vi "Trigger FXP(+,-,18,1).vi"(0 "data A":fxp<+/-,18,1>[](array[numeric])=[0.0, 0.0], 1 "reset":bool, 2 "trigger.ready for reference":bool, 5 "data B":fxp<+/-,18,1>[](array[numeric])=[0.0, 0.0], 7 "input valid":bool, 9 "trigger.A":T9, 11 "trigger.B":T8, 12 "trigger.combination type":T11=enum."A", 13 "rearm delay":u16=2) -> (4 "timestamps":T2, 6 "trigger.out":T10, 8 "overflow":bool, 10 "trigger Source":T1)   [LabVIEW 2021]
uses:
  FPGA Interface Typedefinitions/Trigger Combination Type.ctl
  <instrlib>/_niInstr/Types/v1/Shared/Public/Input Triggers.ctl
  SubVIs/Types/Trigger Type.ctl
  <instrlib>/_niInstr/Data Trigger/v1/Shared/Public/Level Configuration FXP(+-,18,1).ctl
  <instrlib>/_niInstr/Data Trigger/v1/Shared/Public/Level Configuration Trigger When.ctl
  <instrlib>/_niInstr/Data Trigger/v1/Shared/Public/Edge Configuration FXP(+-,18,1).ctl
  <instrlib>/_niInstr/Data Trigger/v1/Shared/Public/Edge Configuration Trigger Slope.ctl
  <instrlib>/_niInstr/Multirecord Acquisition/Interface/v1/FPGA/Public/Timestamp.ctl
  Controls/Clust/TrigSource.ctl
  <instrlib>/_niInstr/Data Trigger/v1/FPGA/Private/Trigger/Level FXP(+-,18,1)xNspc.vi
  <instrlib>/_niInstr/Data Trigger/v1/FPGA/Private/Trigger/Edge FXP(+-,18,1)xNspc.vi
  Trigger Interpolation/Trigger Interpolation FXP(+,-,18,1)x2spc.vi
  <instrlib>/_niInstr/Basic Elements/v1/FPGA/Private/D Latch U16.vi
  <instrlib>/_niInstr/Types/v1/Shared/niInstr Types v1 Shared.lvlib
  <instrlib>/_niInstr/Basic Elements/v1/FPGA/niInstr Basic Elements v1 FPGA.lvlib
  <instrlib>/_niInstr/Data Trigger/v1/FPGA/niInstr Data Trigger v1 FPGA.lvlib
  <instrlib>/_niInstr/Multirecord Acquisition/Interface/v1/FPGA/niInstr Multirecord Acquisition v1 FPGA.lvclass
  <instrlib>/_niInstr/Data Trigger/v1/Shared/niInstr Data Trigger v1 Shared.lvlib
  FPGA Interface Typedefinitions/FPGA Interface Typedefinitions.lvlib
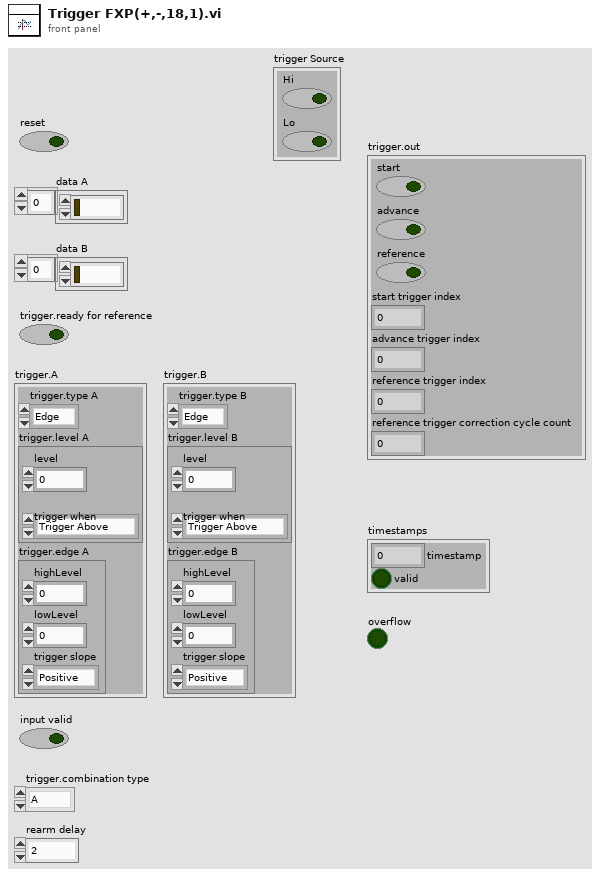
[diagram p1: front panel]
types:
  T1 = typedef "TrigSource.ctl" = cluster{"Hi":bool, "Lo":bool}
  T2 = typedef "niInstr Multirecord Acquisition v1 FPGA.lvclass/Timestamp.ctl" = cluster{"timestamp":u64, "valid":bool}
  T3 = typedef "Trigger Type.ctl" = enum16{"Edge", "Level", "Custom"}
  T4 = typedef "niInstr Data Trigger v1 Shared.lvlib/Level Configuration FXP(+-,18,1).ctl" = cluster{"level":fxp<+/-,18,5>, "trigger when":T5}
  T5 = typedef "niInstr Data Trigger v1 Shared.lvlib/Level Configuration Trigger When.ctl" = enum8{"Trigger Above", "Trigger Below"}
  T6 = typedef "niInstr Data Trigger v1 Shared.lvlib/Edge Configuration FXP(+-,18,1).ctl" = cluster{"highLevel":fxp<+/-,18,1>, "lowLevel":fxp<+/-,18,1>, "trigger slope":T7}
  T7 = typedef "niInstr Data Trigger v1 Shared.lvlib/Edge Configuration Trigger Slope.ctl" = enum8{"Positive", "Negative"}
  T8 = cluster{"trigger.type B":T3, "trigger.level B":T4, "trigger.edge B":T6}
  T9 = cluster{"trigger.type A":T3, "trigger.level A":T4, "trigger.edge A":T6}
  T10 = typedef "niInstr Types v1 Shared.lvlib/Input Triggers.ctl" = cluster{"start":bool, "advance":bool, "reference":bool, "start trigger index":u16, "advance trigger index":u16, "reference trigger index":u16, "reference trigger correction cycle count":u32}
  T11 = typedef "FPGA Interface Typedefinitions.lvlib/Trigger Combination Type.ctl" = enum16{"Immediate", "A", "B", "OR", "AND", "A THEN B", "B THEN A", "High Resolution"}
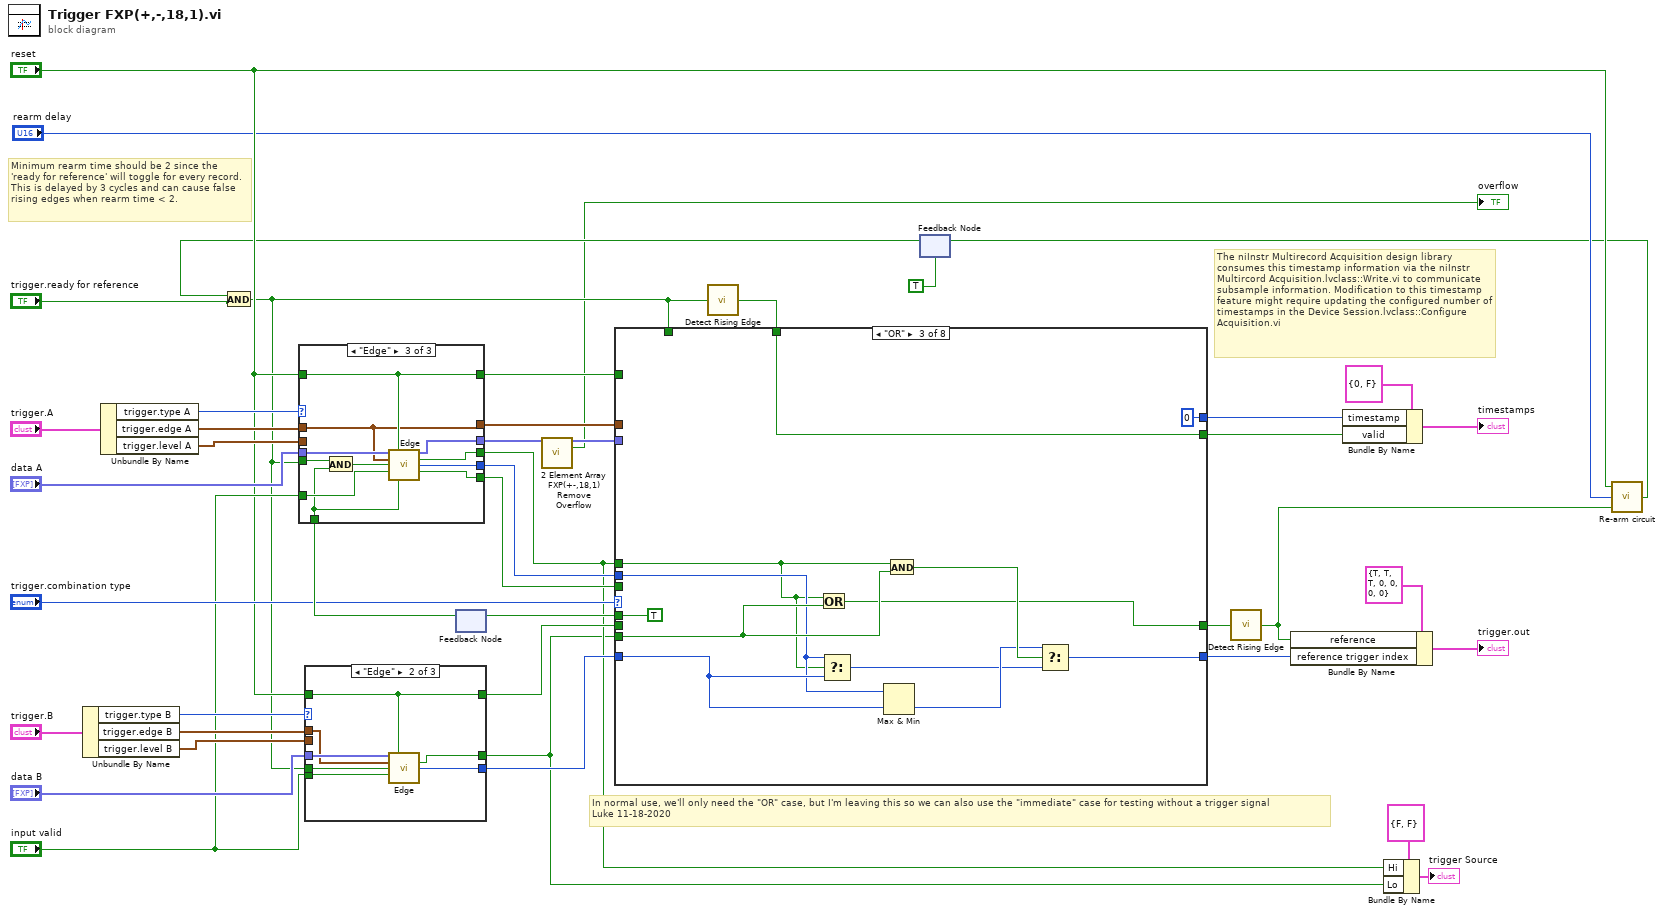
[diagram p0: block diagram]
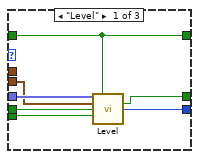
[diagram p2: hidden frame]
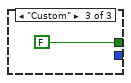
[diagram p3: hidden frame]
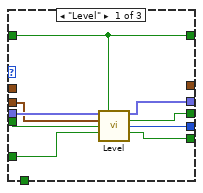
[diagram p4: hidden frame]
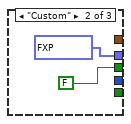
[diagram p5: hidden frame]
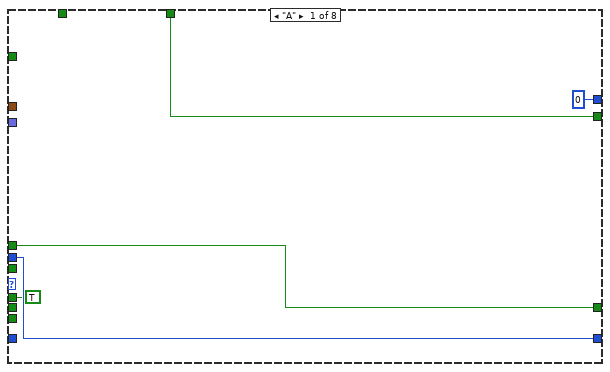
[diagram p6: hidden frame]
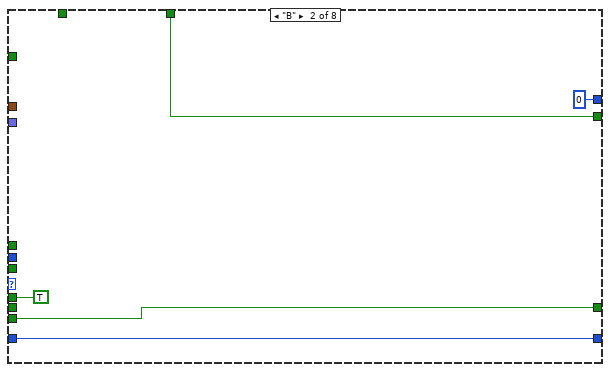
[diagram p7: hidden frame]
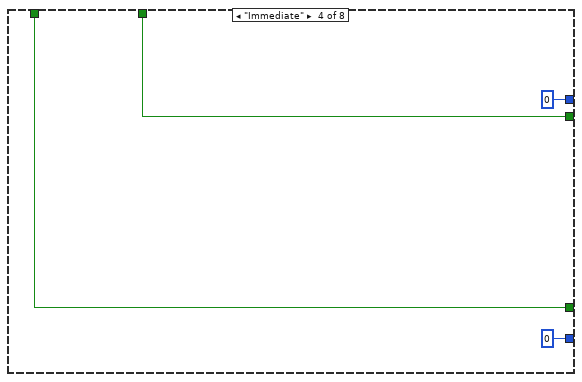
[diagram p8: hidden frame]
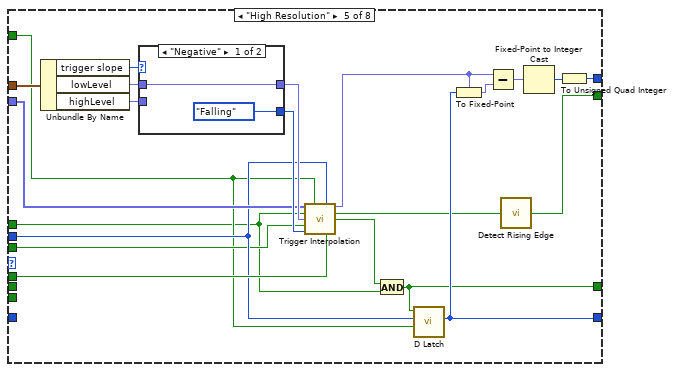
[diagram p9: hidden frame]
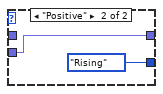
[diagram p10: hidden frame]
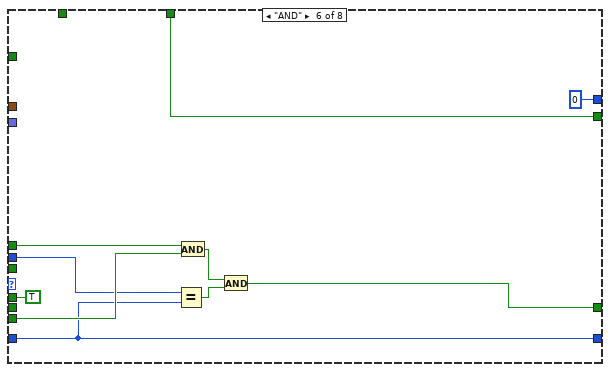
[diagram p11: hidden frame]
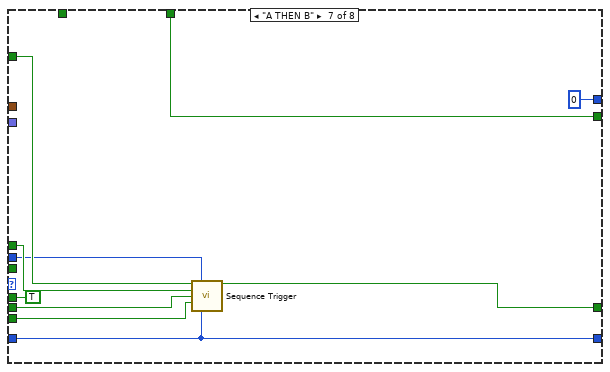
[diagram p12: hidden frame]
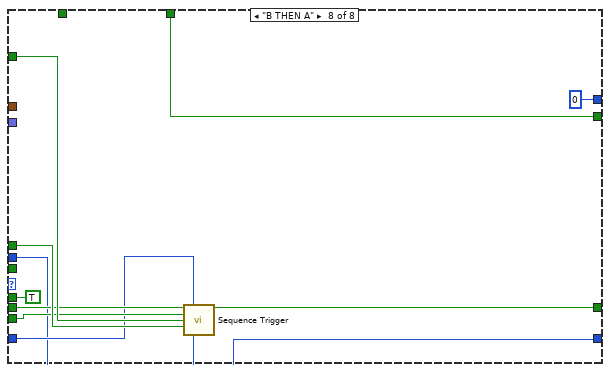
[diagram p13: hidden frame]
diagram:
  # "In normal use, we'll only need the \"OR\" case, but I'm leaving this so we can also use the \"immediate\" case for testing without a trigger signal\nLuke 11-18-2020"
  # "Minimum rearm time should be 2 since the 'ready for reference' will toggle for every record. This is delayed by 3 cycles and can cause false rising edges when rearm time < 2."
  # "The niInstr Multirecord Acquisition design library consumes this timestamp information via the niInstr Multircord Acquisition.lvclass::Write.vi to communicate subsample information. Modification to this timestamp feature might require updating the configured number of timestamps in the Device Session.lvclass::Configure Acquisition.vi"
  n1 = Unbundle By Name("trigger.B") -> ("trigger.type B"=w27:T3, "trigger.edge B"=w25:T6, "trigger.level B"=w26:T4)
  n2 = Unbundle By Name("trigger.A") -> ("trigger.type A"=w28:T3, "trigger.edge A"=w30:T6, "trigger.level A"=w31:T4)
  n3 = feedback #1() -> (w42:bool)  [unwired: 1 in]
  n4 = feedback #2(TRUE ("rearm out")) -> (w9:bool)
  n5 = And(x=w9, y="trigger.ready for reference") -> (x .and. y?=w8:bool)
  n6 = case shown="\"Edge\"" w28 {
    tunnel: "input valid" -> [w53 _ w66]
    tunnel: [w52 FALSE ("trigger") w65] -> w3
    tunnel: [w51 _ w64] -> w35
    tunnel: [w49 _ w62] -> w39
    tunnel: "data A" -> [w50 _ w63]
    tunnel: "reset" -> [w49 _ w62]
    tunnel: [w48 _ w61] -> w41
    tunnel: w8 -> [w46 _ w58]
    tunnel: [_ _ w59] -> w40
    tunnel: [w47 fxp<+/-,18,1>[] [0.0, 0.0] ("data out") w60] -> w7
    tunnel: w42 -> [_ _ w56]
    tunnel: w30 -> [_ _ w59]
    tunnel: w31 -> [w45 _ _]
    frame "Level" {
      n7 = call-poly <instrlib>:"Level.vi"("data in"=w50, "reset"=w49, "configuration"=w45, "arm (T)"=w46, "input valid"=w53) -> ("data out"=w47:fxp<+/-,18,1>[], "trigger"=w52:bool, "trigger index"=w51:u16, "output valid"=w48:bool)  [unwired: 4 in, 3 out]
    }
    frame "Custom" {
    }
    frame "Edge" {
      n8 = And(x=w58, y=w56) -> (x .and. y?=w57:bool)
      n9 = call-poly <instrlib>:"Edge.vi"("data in"=w63, "reset"=w62, "configuration"=w59, "arm (T)"=w57, "input valid"=w66, "ready for output (T)"=w56) -> ("data out"=w60:fxp<+/-,18,1>[], "trigger"=w65:bool, "trigger index"=w64:u16, "output valid"=w61:bool)  [unwired: 4 in, 2 out]
    }
  }
  n10 = case shown="\"Edge\"" w27 {
    tunnel: [w73 w80 FALSE ("trigger")] -> w2
    tunnel: "input valid" -> [w72 w79 _]
    tunnel: [w71 w78 _] -> w36
    tunnel: [w69 w76 _] -> w37
    tunnel: "data B" -> [w70 w77 _]
    tunnel: "reset" -> [w69 w76 _]
    tunnel: w26 -> [w68 _ _]
    tunnel: w25 -> [_ w75 _]
    tunnel: w8 -> [w67 w74 _]
    frame "Level" {
      n11 = call-poly <instrlib>:"Level.vi"("data in"=w70, "reset"=w69, "configuration"=w68, "arm (T)"=w67, "input valid"=w72) -> ("trigger"=w73:bool, "trigger index"=w71:u16)  [unwired: 4 in, 5 out]
    }
    frame "Edge" {
      n12 = call-poly <instrlib>:"Edge.vi"("data in"=w77, "reset"=w76, "configuration"=w75, "arm (T)"=w74, "input valid"=w79) -> ("trigger"=w80:bool, "trigger index"=w78:u16)  [unwired: 5 in, 4 out]
    }
    frame "Custom" {
    }
  }
  n13 = call "2 Element Array FXP(+-,18,1) Remove Overflow.vi"("data in"=w7) -> ("data out"=w6:fxp<+/-,18,1>[], "overflow"=→"overflow":bool)  [unwired: 13 in]
  n14 = call <instrlib>:"Detect Rising Edge.vi"("signal"=w8) -> ("edge detected"=w17:bool)  [unwired: 14 in]
  n15 = case shown="\"OR\"" "trigger.combination type" {
    tunnel: w3 -> [w86 _ w95 _ w110 w143 w152 w161]
    tunnel: w2 -> [_ w91 w97 _ _ w142 w150 w160]
    tunnel: [w86 w91 w94 w105 w108 w138 w149 w163] -> w16
    tunnel: w35 -> [w85 _ w96 _ w115 w141 w145 w154]
    tunnel: w36 -> [_ w90 w98 _ _ w137 w144 w155]
    tunnel: [w85 w90 w93 u16 0 ("trigger index") w117 w137 w144 w154] -> w38
    tunnel: w39 -> [_ _ _ _ w111 _ w153 w162]
    tunnel: w37 -> [_ _ _ _ _ _ w151 w159]
    tunnel: w40 -> [_ _ _ _ w128 _ _ _]
    tunnel: w6 -> [_ _ _ _ w116 _ _ _]
    tunnel: w41 -> [_ _ _ _ w114 _ _ _]
    tunnel: [u64 0 ("trigger time") u64 0 ("trigger time") u64 0 ("trigger time") u64 0 ("trigger time") w126 u64 0 ("trigger time") u64 0 ("trigger time") u64 0 ("trigger time")] -> w24
    tunnel: [w82 w87 w102 w104 w112 w134 w146 w156] -> w23
    tunnel: w8 -> [_ _ _ w105 _ _ _ _]
    tunnel: [TRUE ("ready for input") TRUE ("ready for input") TRUE ("ready for input") _ w124 TRUE ("ready for input") TRUE ("ready for input") TRUE ("ready for input")] -> w43
    tunnel: w17 -> [w82 w87 w102 w104 _ w134 w146 w156]
    frame "A" {
    }
    frame "B" {
    }
    frame "OR" {
      n16 = Or(x=w95, y=w97) -> (x .or. y?=w94:bool)
      n17 = Select(t=w96, s=w95, f=w98) -> (s? t:f=w99:u16)
      n18 = Max & Min(x=w96, y=w98) -> (min(x,y)=w100:u16)  [unwired: 1 out]
      n19 = And(x=w95, y=w97) -> (x .and. y?=w101:bool)
      n20 = Select(t=w100, s=w101, f=w99) -> (s? t:f=w93:u16)
    }
    frame "Immediate" {
    }
    frame "High Resolution" {
      n21 = Unbundle By Name(w128) -> ("trigger slope"=w125:T7, "lowLevel"=w122:fxp<+/-,18,1>, "highLevel"=w121:fxp<+/-,18,1>)
      n22 = case shown="\"Negative\"" w125 {
        tunnel: [enum16{"Rising", "Falling"}."Falling" ("trigger direction") enum16{"Rising", "Falling"}."Rising" ("trigger direction")] -> w129
        tunnel: [w130 w132] -> w123
        tunnel: w122 -> [w130 _]
        tunnel: w121 -> [_ w132]
        frame "Negative" {
        }
        frame "Positive" {
        }
      }
      n23 = call-poly "Trigger Interpolation.vi"("data in"=w116, "reset"=w111, "trigger index"=w115, "trigger"=w110, "trigger level"=w123, "data valid"=w114, "trigger direction"=w129) -> ("trigger time"=w119:fxp<+/-,32,5>, "trigger time valid"=w113:bool, "ready for trigger"=w109:bool, "ready for input"=w124:bool)  [unwired: 4 in, 1 out]
      n24 = And(x=w109, y=w110) -> (x .and. y?=w108:bool)
      n25 = call-poly <instrlib>:"D Latch.vi"("r"=w111, "d"=w115, "s"=w108) -> ("q"=w117:u16)  [unwired: 8 in]
      n26 = To Fixed-Point(fixed-point type=w119, number=w117) -> (fixed-point=w120:fxp<+/-,32,5>)
      n27 = Subtract(x=w119, y=w120) -> (x-y=w118:fxp<+/-,33,6>)
      n28 = call <instrlib>:"Detect Rising Edge.vi"("signal"=w113) -> ("edge detected"=w112:bool)  [unwired: 14 in]
      n29 = Fixed-Point to Integer Cast(1:w118) -> (0:w127:i64)
      n30 = To Unsigned Quad Integer(1:w127) -> (0:w126:u64)
    }
    frame "AND" {
      n31 = Equal?(x=w141, y=w137) -> (x = y?=w139:bool)
      n32 = And(x=w143, y=w142) -> (x .and. y?=w140:bool)
      n33 = And(x=w140, y=w139) -> (x .and. y?=w138:bool)
    }
    frame "A THEN B" {
      n34 = call "Sequence Trigger.vi"("reset A"=w153, "trigger index A"=w145, "A"=w152, "reset B"=w151, "B"=w150, "trigger index B"=w144) -> ("trigger"=w149:bool)  [unwired: 9 in]
    }
    frame "B THEN A" {
      n35 = call "Sequence Trigger.vi"("reset A"=w159, "trigger index A"=w155, "A"=w160, "reset B"=w162, "B"=w161, "trigger index B"=w154) -> ("trigger"=w163:bool)  [unwired: 9 in]
    }
  }
  n36 = feedback-in #1(w43) -> ()
  n37 = call <instrlib>:"Detect Rising Edge.vi"("signal"=w16) -> ("edge detected"=w15:bool)  [unwired: 14 in]
  n38 = Bundle By Name(cluster=T10 {"start"=TRUE, "advance"=TRUE, "reference"=TRUE, "start trigger index"=0, "advance trigger index"=0, "reference trigger index"=0, "reference trigger correction cycle count"=0} ("triggers in"), "reference"=w15, "reference trigger index"=w38) -> (→"trigger.out":T10)
  n39 = Bundle By Name(cluster=T2 {"timestamp"=0, "valid"=FALSE} ("timestamp"), "timestamp"=w24, "valid"=w23) -> (→"timestamps":T2)
  n40 = Bundle By Name(cluster=T1 {"Hi"=FALSE, "Lo"=FALSE} ("TrigSource"), "Hi"=w3, "Lo"=w2) -> (→"trigger Source":T1)
  n41 = call "Re-arm circuit.vi"("trigger"=w15, "delay"="rearm delay", "reset"="reset") -> ("rearm out"=w12:bool)
  n42 = feedback-in #2(w12) -> ()
